vi "IV & Light 2400.vi"() -> ()   [LabVIEW 2017]
uses:
  <vilib>/Utility/file.llb/Write To Spreadsheet File (DBL).vi
panel:
  out "Quantum Efficiency":dbl format="%.4f"
  in  "Stair Voltage":bool=TRUE
  in  "Absolute\nvalue on Plot":bool
  in  "Starting from zero":bool
  out "Number of measurements for negativ Voltage":dbl format="%.2f"
  out "Number of measurements for positiv Voltage":dbl format="%.2f"
  in  "relative (off:0)":i16(slide) scale=0.0..2.0 scale format="%.2f"
  in  "range (auto:0)":i16(slide) scale=0.0..7.0 scale format="%.2f"
  in  "Time Delay(sec) between Pulses\n(Inactive when stairVoltage is ON)":dbl=0.5 format="%.2f"
  in  "Wavelength (nm)":dbl=600.0 format="%.2f"
  in  "Distance (mm) between\nPhoto-and lightemitting Diode":dbl=17.0 format="%.2f"
  out "Sencitivity of Photodiode":dbl=0.4 format="%.2f"
  out "Quantum Efficiency (%)":cluster{dbl[], dbl[]}(graph)
  out "Light vs. Voltage":T1(graph)
  out "Picoamperemeter Current":ext format="%.4e"
  in  "Initilize Array":dbl[](array[numeric]) format="%.2f"
  out "Current vs. Voltage":cluster{dbl[], dbl[]}(graph)
  out "Number of Measurements done":dbl format="%.2f"
  out "Current":dbl format="%.5e"
  in  "range value (amps)":dbl=0.1 min=-3.15 max=3.15 step=5e-11 format="%.3f"
  in  "range (auto:0)":u16(ring)=1 items=["autorange", "set range value"]
  in  "Current Complience":dbl=0.105 format="%.3f"
  in  "Range (Default:0)":u16(ring)=4 items=["Default 20V Range", "Minimum", "Maximum", "By Value", "Auto On", "Auto Off"]
  in  "Time(sec) for stabilisation of current\n(=Puls lenght)":dbl=0.5 format="%.2f"
  in  "stop":bool=TRUE
  out "Start settings":bool=TRUE
  in  "Ending Voltage":dbl format="%.2f"
  in  "Starting Voltage":dbl format="%.2f"
  in  "Increment":dbl=1.0 format="%.2f"
  out "Total Number of measurements":dbl format="%.2f"
  # "I/V & LIGHT Measuring"
  # "FILL IN (input data)"
  # "QE (%)"
  # "%"
  # "Voltage (V)"
  # "Starting from zero = on"
  # "Light (a.u.)"
  # "Current (A)"
  # "Voltage (V)"
  # "Voltage (V)"
  # "NOT NECESSERY TO FILL IN"
  # "Picoamperemeter"
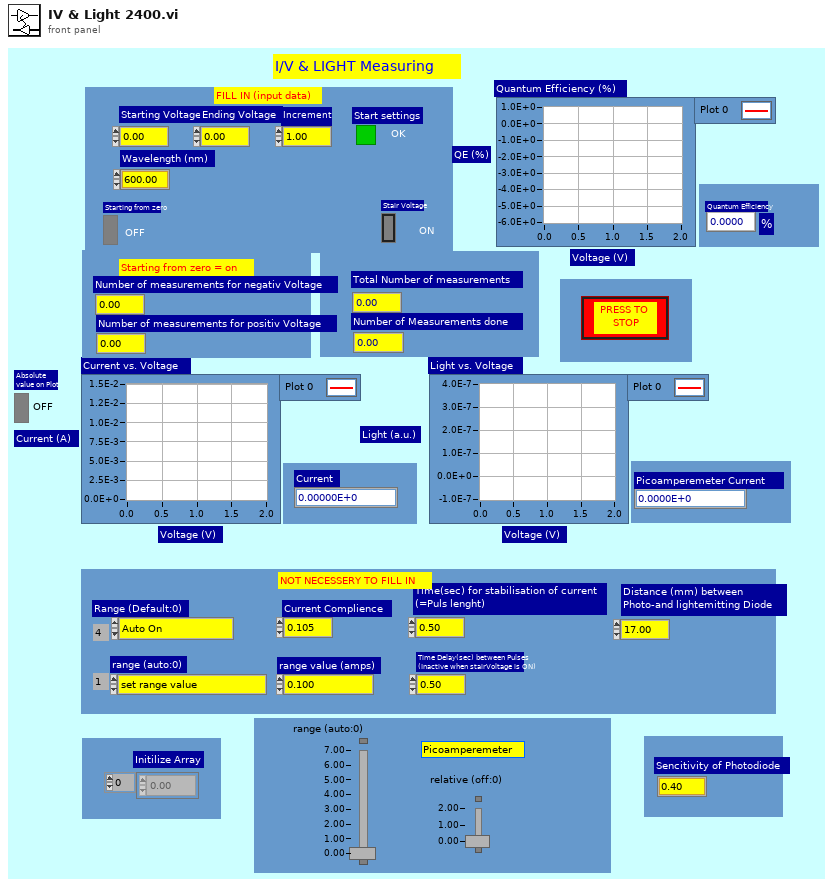
[diagram p1: front panel]
types:
  T1 = cluster{"Output Array":dbl[], "Output Array":dbl[]}
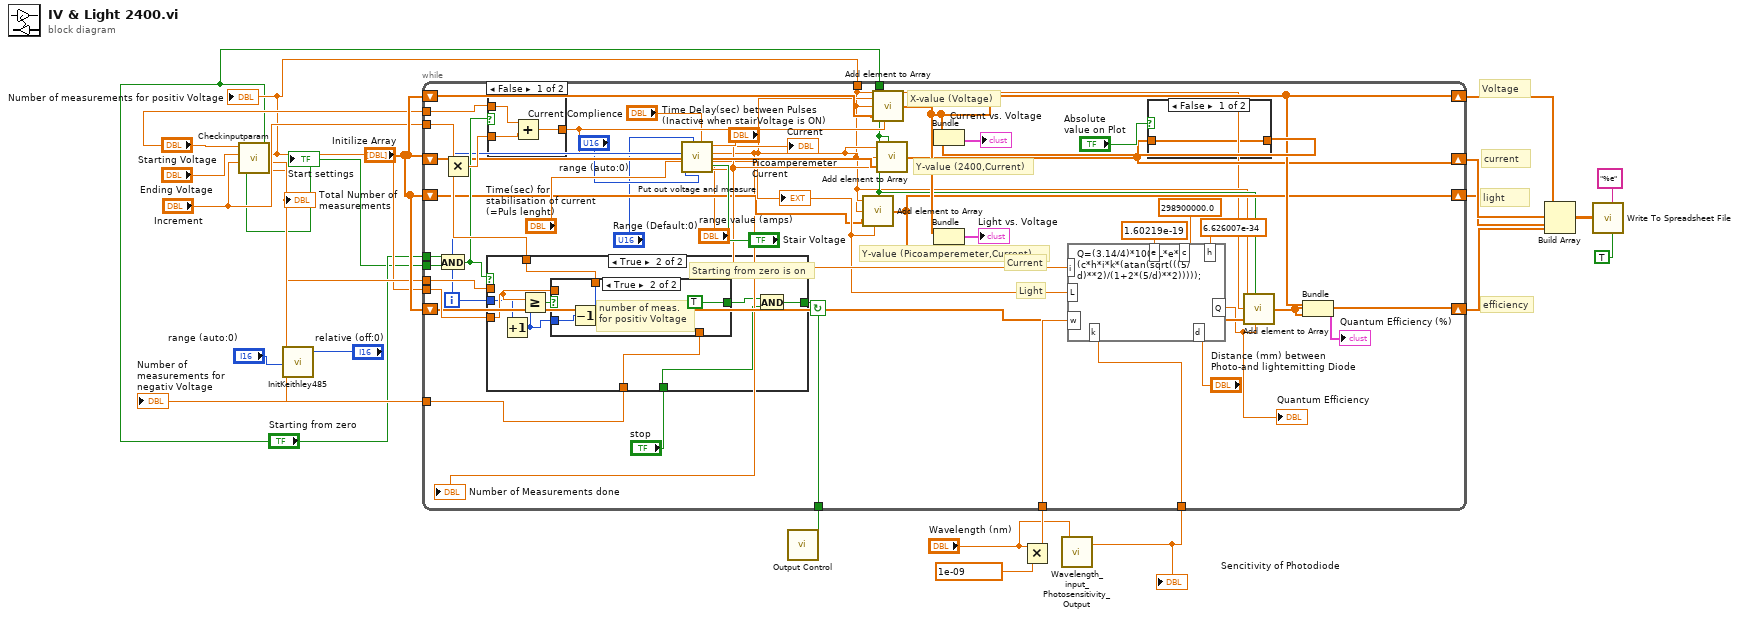
[diagram p0: block diagram]
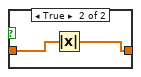
[diagram p2: hidden frame]
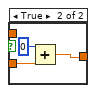
[diagram p3: hidden frame]
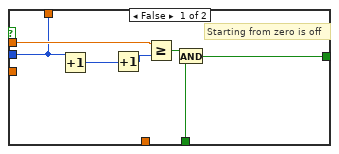
[diagram p4: hidden frame]
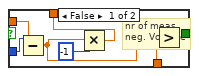
[diagram p5: hidden frame]
diagram:
  # "efficiency"
  # "light"
  # "current"
  # "Voltage"
  n1 = call "Checkinputparam.vi"("Starting from zero"="Starting from zero", "Increment"="Increment", "Ending Voltage"="Ending Voltage", "Starting Voltage"="Starting Voltage") -> ("Number of measurement"=w9:dbl, "Number of measurements for negativ numbers"=w10:dbl, "Number of measurements for positiv numbers"=w3:dbl, "Start settings"=w1:bool)
  "Total Number of measurements" <- w9
  "Start settings" <- w1
  "Number of measurements for positiv Voltage" <- w3
  "Number of measurements for negativ Voltage" <- w10
  n2 = call "InitKeithley485.vi"("range (auto:0)"="range (auto:0)", "relative (off:0)"="relative (off:0)") -> ()  [unwired: 1 in]
  n3 = Multiply(x="Wavelength (nm)", y=1e-09) -> (x*y=w5:dbl)
  n4 = call "Wavelength_input_Photosensitivity_Output.vi"("Wavelength"="Wavelength (nm)") -> ("Sensitivity"=w6:dbl)  [unwired: 1 in]
  "Sencitivity of Photodiode" <- w6
  n5 = while {
    tunnel: "Starting from zero" -> [w31]
    tunnel: w3 -> [w29]
    tunnel: w6 -> [w43]
    tunnel: w5 -> [w44]
    tunnel: w3 -> [w52]
    tunnel: w10 -> [w50]
    tunnel: "Starting from zero" -> [w58]
    tunnel: [w53] -> w8
    shift-left: "Initilize Array" -> [w33]
    shift-right: [w32] -> w18
    shift-left: "Initilize Array" -> [w35]
    shift-right: [w34] -> w19
    shift-left: "Initilize Array" -> [w39]
    shift-right: [w37] -> w20
    shift-left: "Initilize Array" -> [w42]
    shift-right: [w41] -> w21
    tunnel: "Starting Voltage" -> [w57]
    tunnel: "Increment" -> [w69]
    tunnel: w9 -> [w49]
    tunnel: w1 -> [w59]
    i -> [w48]
    stop <- w53 continue-if-true
    # "Light"
    # "Current"
    # "Y-value (Picoamperemeter,Current)"
    # "Y-value (2400,Current)"
    # "X-value (Voltage)"
    n6 = And(x=w58, y=w59) -> (x .and. y?=w51:bool)
    n7 = case shown="True" w51 {
      tunnel: w48 -> [w79 w86]
      tunnel: [w79 w90] -> w61
      tunnel: w49 -> [w83 _]
      tunnel: "stop" -> [w81 w92]
      tunnel: [w82 w91] -> w53
      tunnel: w50 -> [_ w89]
      tunnel: w52 -> [_ w88]
      frame False {
        # "Starting from zero is off"
        n8 = Increment(x=w79) -> (x+1=w80:i32)
        n9 = Increment(x=w80) -> (x+1=w85:i32)
        n10 = Greater Or Equal?(x=w83, y=w85) -> (x >= y?=w84:bool)
        n11 = And(x=w84, y=w81) -> (x .and. y?=w82:bool)
      }
      frame True {
        # "Starting from zero is on"
        n12 = Increment(x=w86) -> (x+1=w87:i32)
        n13 = Greater Or Equal?(x=w88, y=w87) -> (x >= y?=w94:bool)
        n14 = case shown="True" w94 {
          tunnel: w87 -> [w99 w103]
          tunnel: [w100 w102] -> w90
          tunnel: [w96 TRUE] -> w93
          tunnel: w88 -> [w98 _]
          tunnel: w89 -> [w95 _]
          frame False {
            # "nr of meas\nneg. Voltage"
            n15 = Subtract(x=w99, y=w98) -> (x-y=w97:dbl)
            n16 = Multiply(x=w97, y=-1) -> (x*y=w100:dbl)
            n17 = Greater?(x=w95, y=w97) -> (0:w96:bool)
          }
          frame True {
            # "number of meas.\nfor positiv Voltage"
            n18 = Decrement(x=w103) -> (x-1=w102:i32)
          }
        }
        n19 = And(x=w93, y=w92) -> (x .and. y?=w91:bool)
      }
    }
    n20 = Multiply(x=w69, y=w61) -> (x*y=w56:dbl)
    n21 = case shown="False" w51 {
      tunnel: [w75 w76] -> w40
      tunnel: w56 -> [w74 w78]
      tunnel: w57 -> [w73 _]
      frame False {
        n22 = Add(x=w73, y=w74) -> (x+y=w75:dbl)
      }
      frame True {
        n23 = Add(x=0, y=w78) -> (x+y=w76:dbl)
      }
    }
    n24 = call "Put out voltage and measure.vi"("Time Delay between measurements"="Time Delay(sec) between Pulses\n(Inactive when stairVoltage is ON)", "Stair Voltage"="Stair Voltage", "Current Complience"="Current Complience", "range value (amps)"="range value (amps)", "Range (Default:0)"="Range (Default:0)", "range (auto:0)"="range (auto:0)", "Time for current to stabalize before measure the current"="Time(sec) for stabilisation of current\n(=Puls lenght)", "number of interation in the while loop of I/V meas. & Light"=w48, "Output value in volts"=w40) -> ("Reading Result in number"=w38:dbl, "output Picoamperemeter"=w36:ext, "Number of measurements done"=w30:dbl)
    "Current" <- w38
    "Picoamperemeter Current" <- w36
    "Number of Measurements done" <- w30
    n25 = call "Add element to Array.vi"("Number of measurements done"=w30, "Starting from zero"=w31, "Number of measurements for positiv Voltage"=w29, "Array(Current, Light or Voltage)"=w35, "Current , light or Voltage element"=w36) -> ("Output Array"=w34:dbl[])  [unwired: 2 in]
    n26 = call "Add element to Array.vi"("Number of measurements done"=w30, "Starting from zero"=w31, "Number of measurements for positiv Voltage"=w29, "Array(Current, Light or Voltage)"=w42, "Current , light or Voltage element"=w40) -> ("Output Array"=w41:dbl[])  [unwired: 2 in]
    n27 = call "Add element to Array.vi"("Number of measurements done"=w30, "Starting from zero"=w31, "Number of measurements for positiv Voltage"=w29, "Array(Current, Light or Voltage)"=w39, "Current , light or Voltage element"=w38) -> ("Output Array"=w37:dbl[])  [unwired: 2 in]
    n28 = Bundle("Output Array"=w41, "Output Array"=w34) -> (→"Light vs. Voltage":T1)  [unwired: 1 in]
    n29 = formula code="Q=(3.14/4)*100*L*e*w/(c*h*i*k*(atan(sqrt(((5/d)**2)/(1+2*(5/d)**2)))));"("i"=w38, "L"=w36, "k"=w43, "d"="Distance (mm) between\nPhoto-and lightemitting Diode", "w"=w44, "e"=1.60219e-19, "c"=298900000.0, "h"=6.626007e-34) -> ("Q"=w28:dbl)
    "Quantum Efficiency" <- w28
    n30 = case shown="False" "Absolute\nvalue on Plot" {
      tunnel: [w70 w71] -> w54
      tunnel: w37 -> [w70 w72]
      frame False {
      }
      frame True {
        n31 = Absolute Value(x=w72) -> (abs(x)=w71:dbl[])
      }
    }
    n32 = Bundle("Output Array"=w41, "Output Array"=w54) -> (→"Current vs. Voltage":T1)  [unwired: 1 in]
    n33 = call "Add element to Array.vi"("Number of measurements done"=w30, "Starting from zero"=w31, "Number of measurements for positiv Voltage"=w29, "Array(Current, Light or Voltage)"=w33, "Current , light or Voltage element"=w28) -> ("Output Array"=w32:dbl[])  [unwired: 2 in]
    n34 = Bundle("Output Array"=w41, "Output Array"=w32) -> (→"Quantum Efficiency (%)":T1)  [unwired: 1 in]
  }
  n35 = call "Output Control.VI"("Output controller"=w8) -> ()  [unwired: 1 in]
  n36 = Build Array(w21, w20, w19, w18) -> (w16:dbl[][])
  n37 = call-poly <vilib>:"Write To Spreadsheet File.vi"("transpose? (no:F)"=TRUE, "format (%.3f)"="%e", "2D data"=w16) -> ()  [unwired: 5 in, 1 out]
